vi "习3.1.vi"() -> ()   [LabVIEW 2017]
panel:
  out "cosx":dbl
  out "sinx":dbl
  in  "数值":dbl
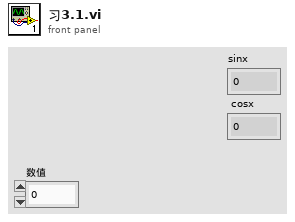
[diagram p1: front panel]
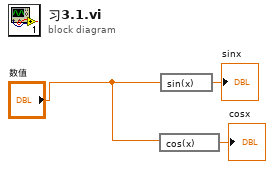
[diagram p0: block diagram]
diagram:
  n1 = expression code="cos(x)"("数值") -> (→"cosx":dbl)
  n2 = expression code="sin(x)"("数值") -> (→"sinx":dbl)
